vi "Limits at zero.vi"() -> (0 "lower limit":dbl, 1 "upper limit":dbl)   [LabVIEW 2014]
uses:
  Labby Bird/Labby Bird/Labby bird-Support.llb/Global-1.vi
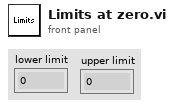
[diagram p1: front panel]
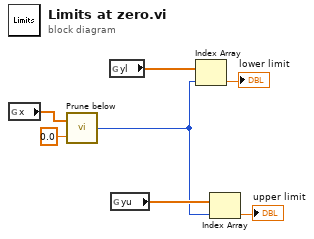
[diagram p0: block diagram]
diagram:
  n1 = global read "Global-1.vi" "x"() -> (w7:dbl[])
  n2 = call "Prune below.vi"("lower limit"=0.0, "Array in"=w7) -> ("Index out"=w1:i32)
  n3 = global read "Global-1.vi" "yl"() -> (w5:dbl[])
  n4 = global read "Global-1.vi" "yu"() -> (w2:dbl[])
  n5 = Index Array(array=w5, index=w1) -> (element=→"lower limit":dbl)
  n6 = Index Array(array=w2, index=w1) -> (element=→"upper limit":dbl)
